vi "XY Graph Delete Plot.vi"(8 "Error In":errorcluster, 9 "Plot Index":i32, 11 "XYGraph Ref":T1) -> (0 "Error Out":errorcluster, 2 "Plot Name":string, 3 "XYGraph Ref":T1, 5 "Graph Caption (or Label)":string)   [LabVIEW 2019, in "XY Graph Add-Ons.lvlib"]
uses:
  XY Graph Add-Ons.lvlib
  XY Graph Refnum.ctl
  Plot Update Steps.ctl
  XY Graph Plot Properties.ctl
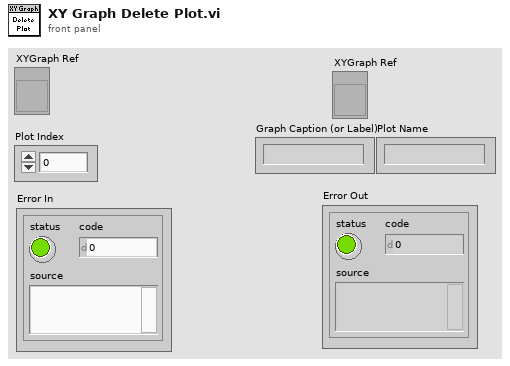
[diagram p1: front panel]
types:
  T1 = typedef "XY Graph Add-Ons.lvlib/XY Graph Refnum.ctl" = refnum<vi>
  T2 = typedef "Plot Update Steps.ctl" = enum16{"Update Plot Styles", "Update Annotation List", "Update Cursor List", "Update Plots", "Quit"}
  T3 = typedef "XY Graph Plot Properties.ctl" = cluster{"Plot Index":i32, "Plot.Bar Plot Style":u8, "Plot.DigitalLineStyle":u8, "Plot.TransitionLocation":u8, "Plot.Transition Type":u8, "Plot.Fill To":i16, "Plot.Fill/Pt. Color":u32, "Plot.Label Format":u8, "Plot.Line Style":u8, "Plot.Line Width":u8, "Plot.Plot Color":u32, "Plot.Plot Interpolation":u8, "Plot.Plot Name":string, "Plot.Point Style":u8, "Plot.Visible?":bool, "Plot.XScaleIdx":u32, "Plot.YScaleIdx":u32, "Plot.Anti-aliased":bool}
  T4 = typedef "LVAnnotationListTypeDef.ctl" = cluster{"Name":string, "Color":u32, "Style":u8, "Point Style":u8, "Name Visible":bool, "Allow Drag":bool, "Annotation Mode":u32, "Plot":i32, "Index":i32, "Position":cluster{"X":dbl, "Y":dbl}, "X Scale":u32, "Y Scale":u32, "Show Arrow":bool, "Lock Name":bool, "Plot Area":i32, "Label Offset":cluster{"X":dbl, "Y":dbl}}[]
  T5 = typedef "LVCursorListTypeDef.ctl" = cluster{"Name":string, "Color":u32, "Style":u8, "Point Style":u8, "Name Visible":bool, "Allow Drag":bool, "Cursor Mode":u32, "Plot":i32, "Index":i32, "Position":cluster{"X":dbl, "Y":dbl}, "X Scale":u32, "Y Scale":u32, "Watch Plots":i32[], "Watch All Plots":bool, "Plot Area":i32, "Label Offset":cluster{"X":dbl, "Y":dbl}}[]
  T6 = cluster{"Name":string, "Color":u32, "Style":u8, "Point Style":u8, "Name Visible":bool, "Allow Drag":bool, "Annotation Mode":u32, "Plot":i32, "Index":i32, "Position":cluster{"X":dbl, "Y":dbl}, "X Scale":u32, "Y Scale":u32, "Show Arrow":bool, "Lock Name":bool, "Plot Area":i32, "Label Offset":cluster{"X":dbl, "Y":dbl}}
  T7 = cluster{"Name":string, "Color":u32, "Style":u8, "Point Style":u8, "Name Visible":bool, "Allow Drag":bool, "Cursor Mode":u32, "Plot":i32, "Index":i32, "Position":cluster{"X":dbl, "Y":dbl}, "X Scale":u32, "Y Scale":u32, "Watch Plots":i32[], "Watch All Plots":bool, "Plot Area":i32, "Label Offset":cluster{"X":dbl, "Y":dbl}}
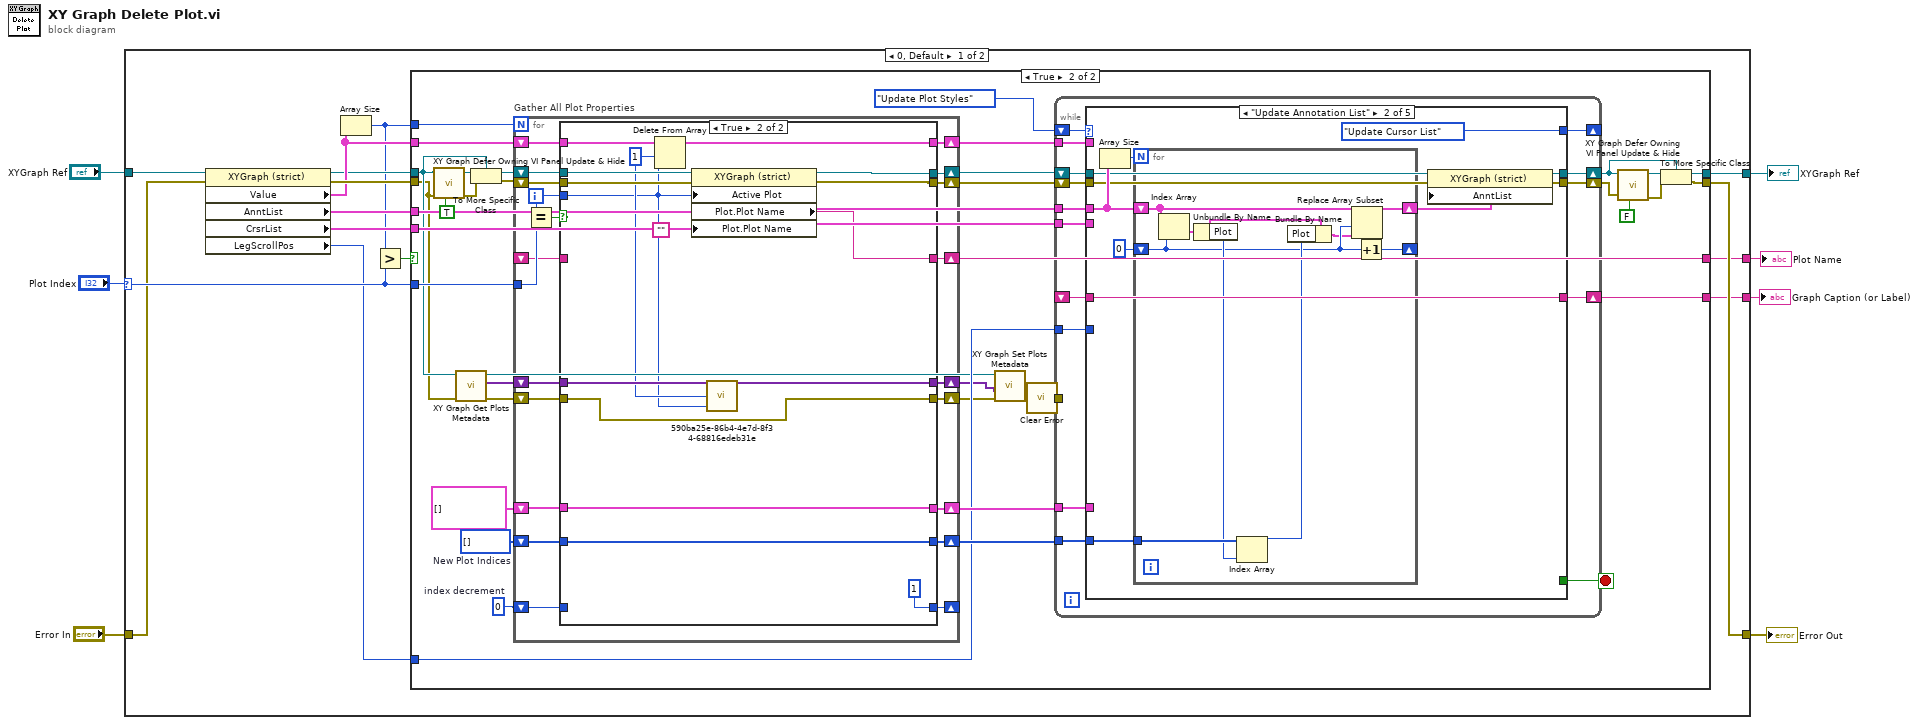
[diagram p0: block diagram]
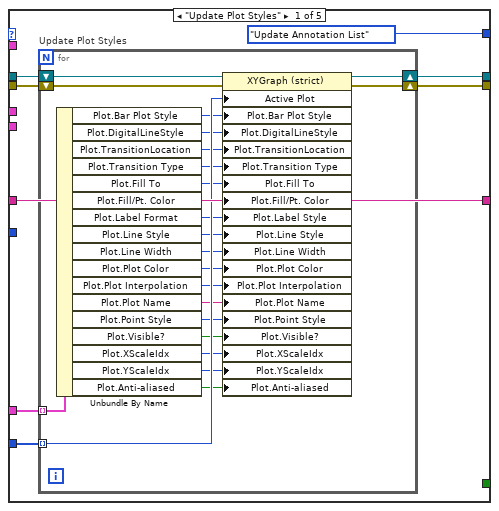
[diagram p3: hidden frame]
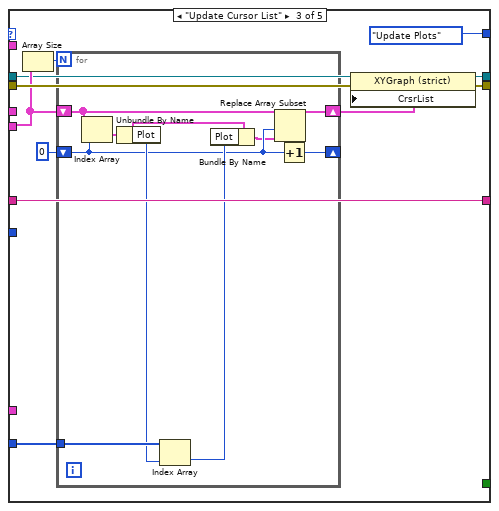
[diagram p4: hidden frame]
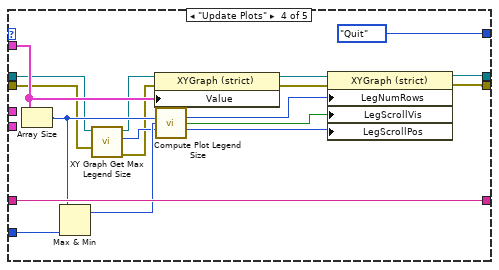
[diagram p5: hidden frame]
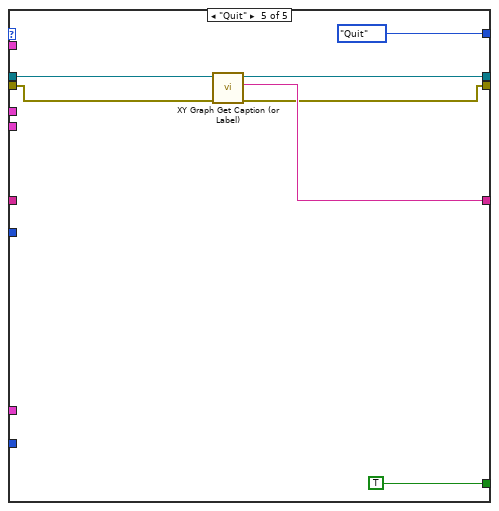
[diagram p6: hidden frame]
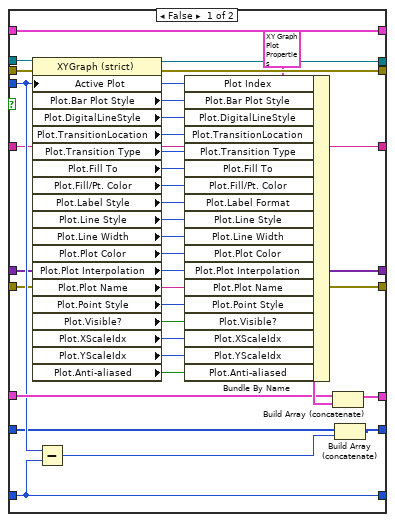
[diagram p7: hidden frame]
diagram:
  n1 = case shown="0, Default" "Plot Index" {
    selector: "Plot Index" -> [w13 _]
    tunnel: "XYGraph Ref" -> [w9 w246]
    tunnel: [w19 w246] -> w5
    tunnel: "Error In" -> [w8 w245]
    tunnel: [w18 w245] -> w3
    tunnel: [w15 _] -> w2
    tunnel: [w14 _] -> w1
    frame 0, Default {
      n2 = property class="XYGraph (strict)"(reference=w9, error in=w8) -> (reference out=w16:T1, error out=w22:errorcluster, "Value"=w21:cluster{"X Array":dbl[], "Y Array":dbl[]}[], "AnntList"=w20:T4, "CrsrList"=w17:T5, "LegScrollPos"=w10:u32)
      n3 = Array Size(array=w21) -> (size(s)=w12:i32)
      n4 = Greater?(x=w12, y=w13) -> (0:w11:bool)
      n5 = case shown="True" w11 {
        tunnel: w22 -> [w23 w32]
        tunnel: w21 -> [_ w61]
        tunnel: w20 -> [_ w55]
        tunnel: [w24 w37] -> w19
        tunnel: [w23 w34] -> w18
        tunnel: w17 -> [_ w53]
        tunnel: w16 -> [w24 w33]
        tunnel: [_ w52] -> w15
        tunnel: [_ w51] -> w14
        tunnel: w13 -> [_ w50]
        tunnel: w12 -> [_ w49]
        tunnel: w10 -> [_ w48]
        frame False {
        }
        frame True {
          w58 = i32[] []  # New Plot Indices
          w60 = 0  # index decrement
          n6 = call "XY Graph Defer Owning VI Panel Update & Hide.vi"("Defer Owning Panel Update"=TRUE, "error in (no error)"=w32, "XY Graph Refnum in"=w33) -> ("error out"=w39:errorcluster, "XY Graph Refnum out"=w41:refnum<vi>)  [unwired: 7 in]
          n7 = call "XY Graph Get Plots Metadata.vi"("Error In"=w32, "XYGraph Ref"=w33) -> ("Error Out"=w31:errorcluster, "Plots Metadata"=w30:variant[], "XYGraph Ref (dup)"=w26:T1)  [unwired: 6 in, 1 out]
          n8 = To More Specific Class(target class=w33, reference=w41, error in=w39) -> (specific class reference=w40:T1, error out=w38:errorcluster)
          n9 = for "Gather All Plot Properties" {
            N: w49 -> [_]
            tunnel: w50 -> [w192]
            shift-right: [w189] -> w54
            shift-left: w61 -> [w190]
            shift-right: [w184] -> w59
            shift-left: T3[] [] -> [w185]
            shift-right: [w186] -> w46
            shift-left: w38 -> [w187]
            shift-right: [w182] -> _
            shift-left: w60 -> [w183]
            shift-right: [w180] -> w57
            shift-left: w58 -> [w181]
            shift-right: [w188] -> w47
            shift-left: w40 -> [w194]
            shift-right: [w179] -> w51
            shift-left: _ -> [w178]
            shift-right: [w176] -> w29
            shift-left: w31 -> [w177]
            shift-right: [w174] -> w25
            shift-left: w30 -> [w175]
            i -> [w193]
            n10 = Equal?(x=w193, y=w192) -> (x = y?=w191:bool)
            n11 = case shown="True" w191 {
              tunnel: w194 -> [w228 w242]
              tunnel: w193 -> [w203 w231]
              tunnel: w190 -> [w227 w244]
              tunnel: [w227 w243] -> w189
              tunnel: [w226 w238] -> w188
              tunnel: w187 -> [w225 w237]
              tunnel: [w224 w236] -> w186
              tunnel: w185 -> [w205 w241]
              tunnel: [w204 w241] -> w184
              tunnel: w183 -> [w202 _]
              tunnel: [w202 1 ("index decrement")] -> w182
              tunnel: w181 -> [w201 w239]
              tunnel: [w199 w239] -> w180
              tunnel: [w198 w235] -> w179
              tunnel: w178 -> [w198 _]
              tunnel: w177 -> [w196 w229]
              tunnel: [w196 w229] -> w176
              tunnel: w175 -> [w195 w233]
              tunnel: [w195 w230] -> w174
              frame False {
                n12 = property class="XYGraph (strict)"(reference=w228, error in=w225, "Active Plot"=w203) -> (reference out=w226:T1, error out=w224:errorcluster, "Plot.Bar Plot Style"=w223:u8, "Plot.DigitalLineStyle"=w222:u8, "Plot.TransitionLocation"=w221:u8, "Plot.Transition Type"=w220:u8, "Plot.Fill To"=w219:i16, "Plot.Fill/Pt. Color"=w218:u32, "Plot.Label Style"=w217:u8, "Plot.Line Style"=w216:u8, "Plot.Line Width"=w215:u8, "Plot.Plot Color"=w214:u32, "Plot.Plot Interpolation"=w213:u8, "Plot.Plot Name"=w212:string, "Plot.Point Style"=w211:u8, "Plot.Visible?"=w210:bool, "Plot.XScaleIdx"=w209:u32, "Plot.YScaleIdx"=w208:u32, "Plot.Anti-aliased"=w197:bool)
                n13 = Subtract(x=w203, y=w202) -> (x-y=w200:i32)
                n14 = Bundle By Name(cluster=T3 {"Plot Index"=0, "Plot.Bar Plot Style"=0, "Plot.DigitalLineStyle"=0, "Plot.TransitionLocation"=0, "Plot.Transition Type"=0, "Plot.Fill To"=0, "Plot.Fill/Pt. Color"=0, "Plot.Label Format"=0, "Plot.Line Style"=0, "Plot.Line Width"=0, "Plot.Plot Color"=0, "Plot.Plot Interpolation"=0, "Plot.Plot Name"="", "Plot.Point Style"=0, "Plot.Visible?"=FALSE, "Plot.XScaleIdx"=0, "Plot.YScaleIdx"=0, "Plot.Anti-aliased"=FALSE}, "Plot Index"=w203, "Plot.Bar Plot Style"=w223, "Plot.DigitalLineStyle"=w222, "Plot.TransitionLocation"=w221, "Plot.Transition Type"=w220, "Plot.Fill To"=w219, "Plot.Fill/Pt. Color"=w218, "Plot.Label Format"=w217, "Plot.Line Style"=w216, "Plot.Line Width"=w215, "Plot.Plot Color"=w214, "Plot.Plot Interpolation"=w213, "Plot.Plot Name"=w212, "Plot.Point Style"=w211, "Plot.Visible?"=w210, "Plot.XScaleIdx"=w209, "Plot.YScaleIdx"=w208, "Plot.Anti-aliased"=w197) -> (w206:T3)
                n15 = Build Array (concatenate)(w205, w206) -> (w204:T3[])
                n16 = Build Array (concatenate)(w201, w200) -> (w199:i32[])
              }
              frame True {
                w232 = 1 ("length")
                n17 = Delete From Array(array=w244, length=w232, index=w231) -> (array with subset deleted=w243:cluster{"X Array":dbl[], "Y Array":dbl[]}[])  [unwired: 1 out]
                n18 = property class="XYGraph (strict)"(reference=w242, error in=w237, "Active Plot"=w231, "Plot.Plot Name"="") -> (reference out=w238:T1, error out=w236:errorcluster, "Plot.Plot Name"=w235:string)
                n19 = call "590ba25e-86b4-4e7d-8f34-68816edeb31e.vi"("index (last elem)"=w231, "length (1)"=w232, "Array"=w233) -> ("array w/ subset deleted"=w230:variant[])  [unwired: 1 out]
              }
            }
          }
          n20 = call "XY Graph Set Plots Metadata.vi"("error in (no error)"=w29, "Plots Metadata"=w25, "XY Graph Refnum"=w26) -> ("error out"=w28:errorcluster)  [unwired: 7 in, 1 out]
          n21 = call "Clear Error.vi"("Error In"=w28) -> ("no Error Out"=w27:errorcluster)  [unwired: 8 in]
          n22 = while {
            tunnel: w59 -> [w77]
            tunnel: w57 -> [w74]
            shift-right: [w71] -> _
            shift-left: Plot_Update_Steps."Update Plot Styles" -> [w73]
            shift-right: [w63] -> w43
            shift-left: w46 -> [w75]
            tunnel: w55 -> [w70]
            tunnel: w54 -> [w69]
            tunnel: w53 -> [w68]
            shift-right: [w64] -> w36
            shift-left: w47 -> [w76]
            shift-right: [w67] -> w52
            shift-left: _ -> [w66]
            tunnel: w48 -> [w65]
            tunnel: w27 -> [_]
            stop <- w72 stop-if-true
            n23 = case shown="\"Update Annotation List\"" w73 {
              tunnel: w77 -> [w85 _ _ _ _]
              tunnel: w76 -> [w84 w114 w129 w151 w172]
              tunnel: w75 -> [w83 w112 w134 w149 w168]
              tunnel: [w82 w111 w133 w162 w167] -> w63
              tunnel: [w81 w113 w135 w163 w169] -> w64
              tunnel: w74 -> [w80 w118 w138 _ _]
              tunnel: [_ _ _ _ TRUE] -> w72
              tunnel: [Plot_Update_Steps."Update Annotation List" Plot_Update_Steps."Update Cursor List" Plot_Update_Steps."Update Plots" Plot_Update_Steps."Quit" Plot_Update_Steps."Quit"] -> w71
              tunnel: w70 -> [_ w117 _ _ _]
              tunnel: w69 -> [_ _ _ w165 _]
              tunnel: w68 -> [_ _ w131 _ _]
              tunnel: [w78 w109 w130 w160 w170] -> w67
              tunnel: w66 -> [w78 w109 w130 w160 _]
              tunnel: w65 -> [_ _ _ w158 _]
              frame "Update Plot Styles" {
                n24 = for "Update Plot Styles" {
                  tunnel: w85 -> [w108] mode=indexing
                  shift-right: [w104] -> w82
                  shift-left: w83 -> [w105]
                  tunnel: w80 -> [w103] mode=indexing
                  shift-right: [w106] -> w81
                  shift-left: w84 -> [w107]
                  n25 = Unbundle By Name(w108) -> ("Plot.Bar Plot Style"=w102:u8, "Plot.DigitalLineStyle"=w101:u8, "Plot.TransitionLocation"=w100:u8, "Plot.Transition Type"=w99:u8, "Plot.Fill To"=w98:i16, "Plot.Fill/Pt. Color"=w97:u32, "Plot.Label Format"=w96:u8, "Plot.Line Style"=w95:u8, "Plot.Line Width"=w94:u8, "Plot.Plot Color"=w93:u32, "Plot.Plot Interpolation"=w92:u8, "Plot.Plot Name"=w91:string, "Plot.Point Style"=w90:u8, "Plot.Visible?"=w89:bool, "Plot.XScaleIdx"=w88:u32, "Plot.YScaleIdx"=w87:u32, "Plot.Anti-aliased"=w86:bool)
                  n26 = property class="XYGraph (strict)"(reference=w107, error in=w105, "Active Plot"=w103, "Plot.Bar Plot Style"=w102, "Plot.DigitalLineStyle"=w101, "Plot.TransitionLocation"=w100, "Plot.Transition Type"=w99, "Plot.Fill To"=w98, "Plot.Fill/Pt. Color"=w97, "Plot.Label Style"=w96, "Plot.Line Style"=w95, "Plot.Line Width"=w94, "Plot.Plot Color"=w93, "Plot.Plot Interpolation"=w92, "Plot.Plot Name"=w91, "Plot.Point Style"=w90, "Plot.Visible?"=w89, "Plot.XScaleIdx"=w88, "Plot.YScaleIdx"=w87, "Plot.Anti-aliased"=w86) -> (reference out=w106:T1, error out=w104:errorcluster)
                }
              }
              frame "Update Annotation List" {
                n27 = Array Size(array=w117) -> (size(s)=w116:i32)
                n28 = for {
                  N: w116 -> [_]
                  tunnel: w118 -> [w128]
                  shift-right: [w122] -> w110
                  shift-left: w117 -> [w124]
                  shift-right: [w121] -> _
                  shift-left: 0 -> [w123]
                  n29 = Index Array(array=w124, index=w123) -> (element=w126:T6)
                  n30 = Unbundle By Name(w126) -> ("Plot"=w127:i32)
                  n31 = Index Array(array=w128, index=w127) -> (element=w125:i32)
                  n32 = Bundle By Name(cluster=w126, "Plot"=w125) -> (w120:T6)
                  n33 = Replace Array Subset(array=w124, new element=w120, index=w123) -> (w122:T4)
                  n34 = Increment(x=w123) -> (x+1=w121:i32)
                }
                n35 = property class="XYGraph (strict)"(reference=w114, error in=w112, "AnntList"=w110) -> (reference out=w113:T1, error out=w111:errorcluster)
              }
              frame "Update Cursor List" {
                n36 = Array Size(array=w131) -> (size(s)=w137:i32)
                n37 = for {
                  N: w137 -> [_]
                  tunnel: w138 -> [w148]
                  shift-right: [w142] -> w132
                  shift-left: w131 -> [w144]
                  shift-right: [w141] -> _
                  shift-left: 0 -> [w143]
                  n38 = Index Array(array=w144, index=w143) -> (element=w146:T7)
                  n39 = Unbundle By Name(w146) -> ("Plot"=w147:i32)
                  n40 = Index Array(array=w148, index=w147) -> (element=w145:i32)
                  n41 = Bundle By Name(cluster=w146, "Plot"=w145) -> (w140:T7)
                  n42 = Replace Array Subset(array=w144, new element=w140, index=w143) -> (w142:T5)
                  n43 = Increment(x=w143) -> (x+1=w141:i32)
                }
                n44 = property class="XYGraph (strict)"(reference=w129, error in=w134, "CrsrList"=w132) -> (reference out=w135:T1, error out=w133:errorcluster)
              }
              frame "Update Plots" {
                n45 = Array Size(array=w165) -> (size(s)=w157:i32)
                n46 = Max & Min(x=w157, y=w158) -> (max(x,y)=w159:u32)  [unwired: 1 out]
                n47 = call "XY Graph Get Max Legend Size.vi"("Error In"=w149, "XYGraph Refnum"=w151) -> ("Error Out"=w150:errorcluster, "Max Legend Size"=w153:i32, "XYGraph Refnum"=w152:T1)  [unwired: 6 in, 1 out]
                n48 = property class="XYGraph (strict)"(reference=w152, error in=w150, "Value"=w165) -> (reference out=w164:T1, error out=w161:errorcluster)
                n49 = call "Compute Plot Legend Size.vi"("# Plots"=w157, "Current Plot (Last)"=w159, "Max Legend Size"=w153) -> ("LegNumRows"=w156:u32, "LegScrollVis"=w155:bool, "LegScrollPos"=w154:u32)  [unwired: 10 in]
                n50 = property class="XYGraph (strict)"(reference=w164, error in=w161, "LegNumRows"=w156, "LegScrollVis"=w155, "LegScrollPos"=w154) -> (reference out=w163:T1, error out=w162:errorcluster)
              }
              frame "Quit" {
                n51 = call "XY Graph Get Caption (or Label).vi"("error in (no error)"=w168, "XYGraph in"=w172) -> ("error out"=w167:errorcluster, "Caption (or Label) Text"=w170:string, "XYGraph out"=w169:T1)  [unwired: 7 in]
              }
            }
          }
          n52 = call "XY Graph Defer Owning VI Panel Update & Hide.vi"("Defer Owning Panel Update"=FALSE, "error in (no error)"=w43, "XY Graph Refnum in"=w36) -> ("error out"=w35:errorcluster, "XY Graph Refnum out"=w44:refnum<vi>)  [unwired: 7 in]
          n53 = To More Specific Class(target class=w36, reference=w44, error in=w35) -> (specific class reference=w37:T1, error out=w34:errorcluster)
        }
      }
    }
    frame ..-1 {
    }
  }
  "XYGraph Ref" <- w5
  "Error Out" <- w3
  "Graph Caption (or Label)" <- w2
  "Plot Name" <- w1
